vi "Command Drive Time with IMU.vi"(2 "Robot System Functions In":T1, 3 "Startup":bool, 4 "String Parameter":string, 5 "Cmd Parameter 3":dbl, 6 "Cmd Parameter 2":dbl, 7 "Cmd Parameter 1":dbl) -> (0 "Robot System Functions Out":T1, 1 "Completed":bool)   [LabVIEW 2016]
uses:
  Subsystems/All Robot Commands.ctl
  Subsystems/Drive and Climb SS/Drive + Climb Commands 2017.ctl
  Subsystems/Gear Delivery SS/Gear Delivery Commands.ctl
  Subsystems/Conveyor and Shooter SS/Conveyor and Shooter Commands.ctl
  Subsystems/Ball Intake SS/Ball Intake Commands.ctl
  Command Execution State.ctl
  <vilib>/Rock Robotics/WPI/ThirdParty/Sensors/Pigeon IMU/CTRE_PigeonIMU_TareType.ctl
  <vilib>/Rock Robotics/WPI/ThirdParty/CanMotor/TalonSRX/WPI_CANTalonSRX_APIControlMode.ctl
  Global Variables/Refnum Names.vi
  Global Variables/Auto Drive Calibrations.vi
  Global Variables/Sensor Data.vi
panel:
  out "Right F":dbl
  out "Right D":dbl
  out "Right I":dbl
  out "Right P":dbl
  out "Left F":dbl
  out "Left D":dbl
  out "Left I":dbl
  out "Left P":dbl
  # "Sample robot\ncontrol output.\nReplace with \nactual teleop \ncontrol signal \nstructure."
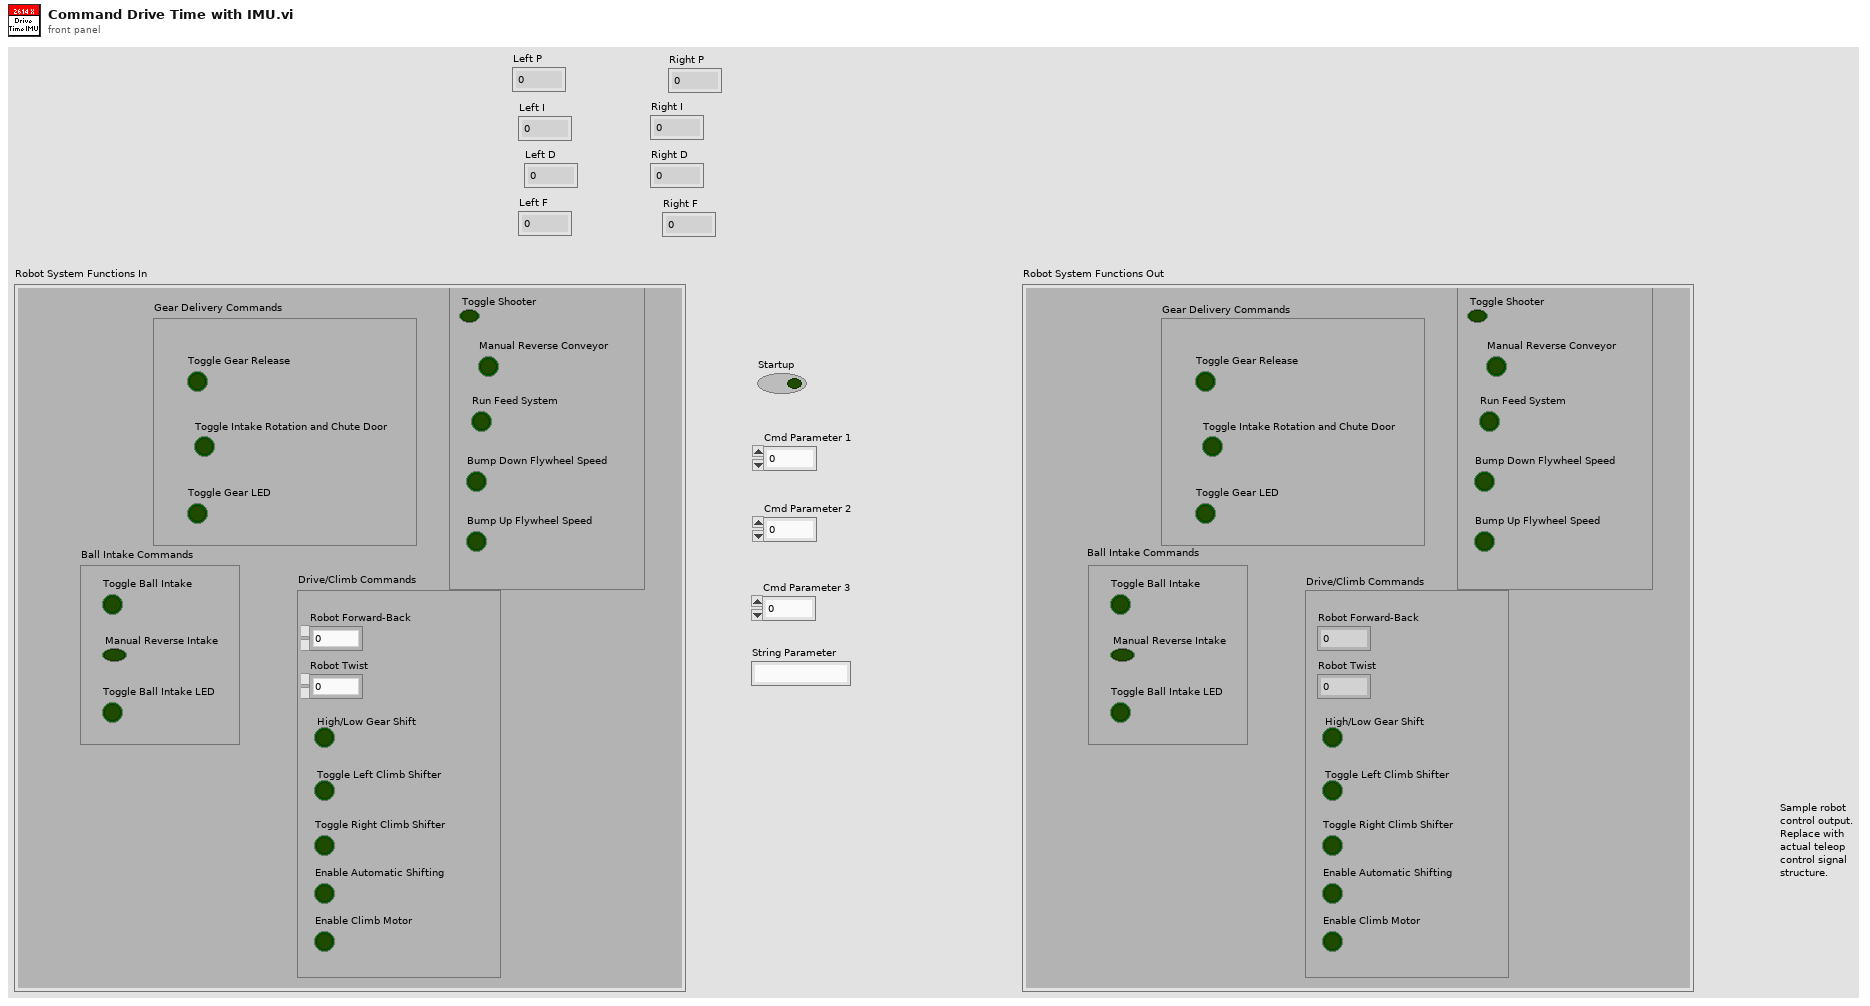
[diagram p1: front panel]
types:
  T1 = typedef "All Robot Commands.ctl" = cluster{"Drive/Climb Commands":T2, "Gear Delivery Commands":T3, "Shooter and Conveyor Commands":T4, "Ball Intake Commands":T5}
  T2 = typedef "Drive + Climb Commands 2017.ctl" = cluster{"Robot Forward-Back":dbl, "Robot Twist":dbl, "High/Low Gear Shift":bool, "Toggle Left Climb Shifter":bool, "Toggle Right Climb Shifter":bool, "Enable Automatic Shifting":bool, "Enable Climb Motor ":bool}
  T3 = typedef "Gear Delivery Commands.ctl" = cluster{"Toggle Gear Release":bool, "Toggle Intake Rotation and Chute Door":bool, "Toggle Gear LED":bool}
  T4 = typedef "Conveyor and Shooter Commands.ctl" = cluster{"Toggle Shooter":bool, "Manual Reverse Conveyor":bool, "Run Feed System":bool, "Bump Down Flywheel Speed":bool, "Bump Up Flywheel Speed":bool}
  T5 = typedef "Ball Intake Commands.ctl" = cluster{"Toggle Ball Intake":bool, "Manual Reverse Intake":bool, "Toggle Ball Intake LED":bool}
  T6 = typedef "Command Execution State.ctl" = enum16{"Initialize", "Execute", "Finish"}
  T7 = typedef "WPI_CANTalonSRX_APIControlMode.ctl" = enum8{"Percent VBus", "Speed", "Position", "Slave", "Unchanged / Invalid", "Voltage Compensation", "Current", "Motion Profile", "Motion Magic"}
  T8 = typedef "CTRE_PigeonIMU_TareType.ctl" = u8
  T9 = typedef "CTRE_PigeonIMU_DeviceRef.ctl" = cluster{"DeviceStatus":errorcluster, "Device Number":u8, "Type":T10, "Device ID":u32}
  T10 = typedef "CTRE_PigeonIMU_ConnectionType.ctl" = u32
  T11 = typedef "WPI_MotorControlDeviceRef.ctl" = cluster{"DeviceStatus":errorcluster, "Type":T12, "PWM":cluster{"PWM Channel":T13, "DeadBand":T14}, "CAN":cluster{"Device Number":u8, "SetOutput VI Ref":variant, "GetOutput VI Ref":variant, "Enable VI Ref":variant, "Disable VI Ref":variant, "Data":variant}, "Invert":bool}
  T12 = typedef "WPI_MotorControlType.ctl" = enum16{"PWM", "CAN"}
  T13 = typedef "FPGA_DIOPWMChannel.ctl" = enum8{"PWM 0", "PWM 1", "PWM 2", "PWM 3", "PWM 4", "PWM 5", "PWM 6", "PWM 7", "PWM 8", "PWM 9", "PWM MXP 0", "PWM MXP 1", "PWM MXP 2", "PWM MXP 3", "PWM MXP 4", "PWM MXP 5", "PWM MXP 6", "PWM MXP 7", "PWM MXP 8", "PWM MXP 9", "Invalid"}
  T14 = typedef "WPI_PWMDeadband.ctl" = cluster{"Name":string, "maxPositivePwm":i32, "minPositivePwm":i32, "centerPwm":i32, "maxNegativePwm":i32, "minNegativePwm":i32, "angularRange":u16}
  T15 = cluster{"Goal":dbl, "Process Variable":dbl, "Max Ouput":dbl, dbl, dbl, dbl, dbl}
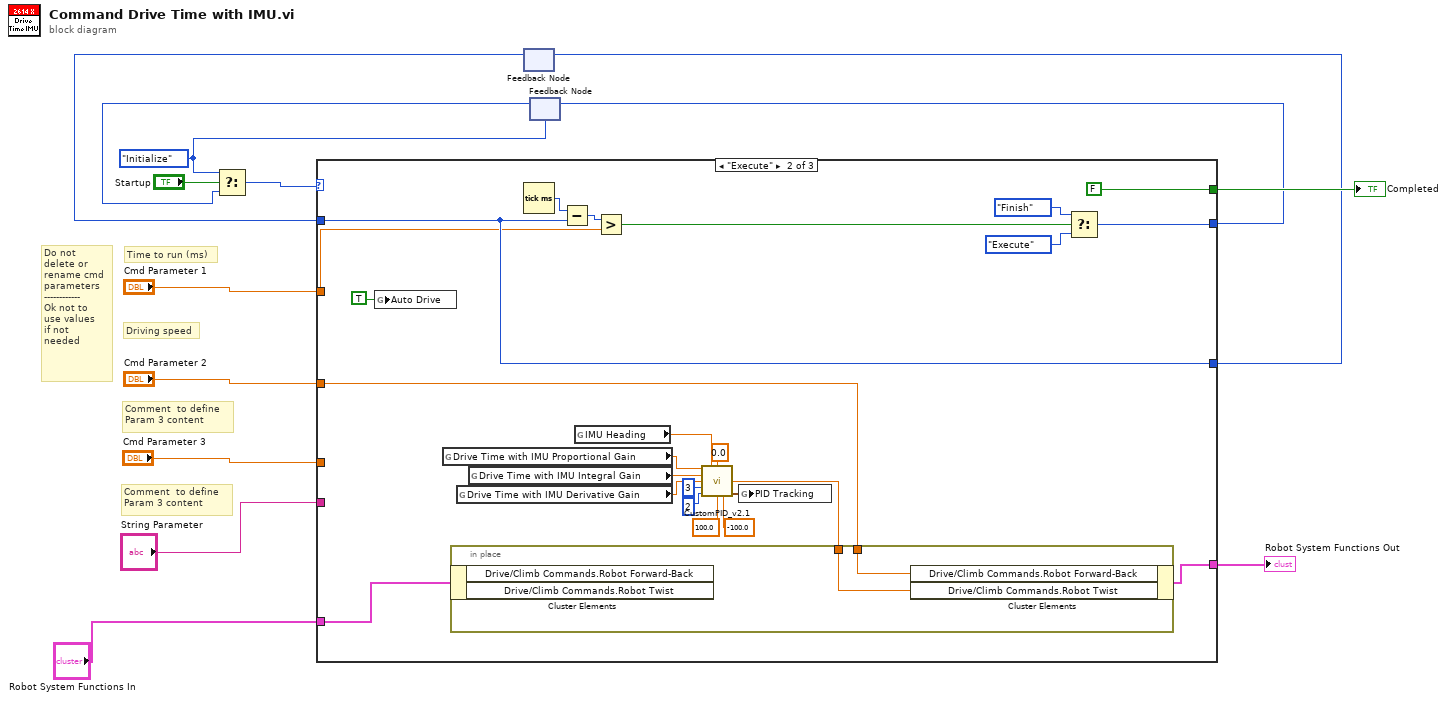
[diagram p0: block diagram]
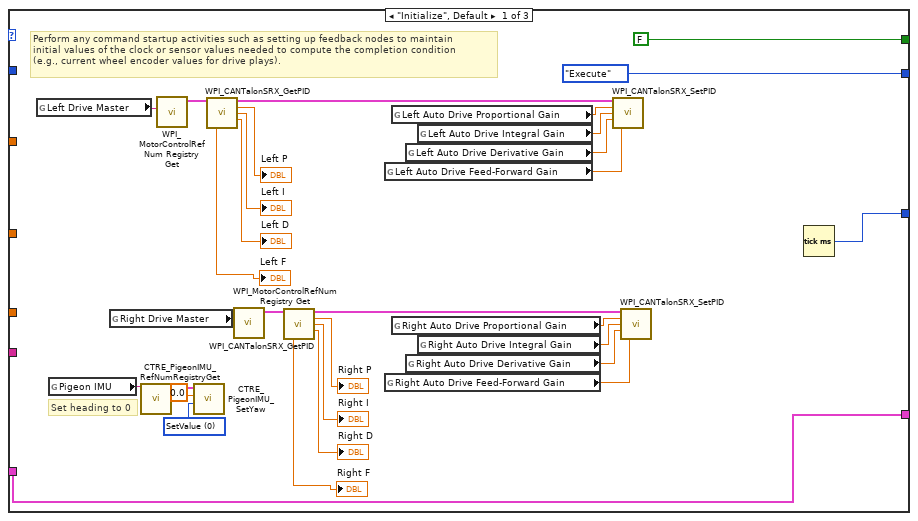
[diagram p2: hidden frame]
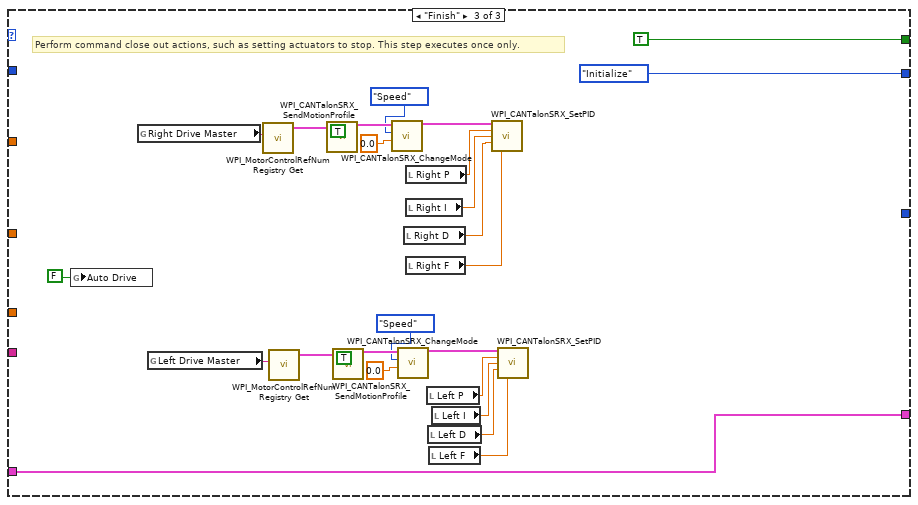
[diagram p3: hidden frame]
diagram:
  w9 = Command_Execution_State."Initialize" ("Play State")
  # "Comment  to define\nParam 3 content"
  # "Comment  to define\nParam 3 content"
  # "Do not \ndelete or\nrename cmd\nparameters\n------------\nOk not to \nuse values\nif not \nneeded"
  # "Driving speed"
  # "Time to run (ms)"
  n1 = feedback #1() -> (w1:u32)  [unwired: 1 in]
  n2 = feedback #2(w9) -> (w10:T6)
  n3 = Select(t=w9, s="Startup", f=w10) -> (s? t:f=w14:T6)
  n4 = case shown="\"Execute\"" w14 {
    tunnel: [FALSE FALSE TRUE] -> w12
    tunnel: [Command_Execution_State."Execute" ("Play State") w66 Command_Execution_State."Initialize" ("f")] -> w11
    tunnel: "Cmd Parameter 1" -> [_ w60 _]
    tunnel: "Cmd Parameter 2" -> [_ w45 _]
    tunnel: [w42 w58 w94] -> w6
    tunnel: "Robot System Functions In" -> [w42 w64 w94]
    tunnel: "Cmd Parameter 3" -> [_ _ _]
    tunnel: "String Parameter" -> [_ _ _]
    tunnel: [w41 w62 _] -> w2
    tunnel: w1 -> [_ w62 _]
    frame "Initialize", Default {
      w27 = T8 0 items=["SetValue"=0, "AddOffset"=1, "MatchCompass"=2, "SetOffset"=255] ("TareType (SetValue)")
      # "Set heading to 0"
      # "Perform any command startup activities such as setting up feedback nodes to maintain \ninitial values of the clock or sensor values needed to compute the completion condition\n(e.g., current wheel encoder values for drive plays)."
      n5 = global read "Refnum Names.vi" "Left Drive Master"() -> (w40:string)
      n6 = global read "Refnum Names.vi" "Pigeon IMU"() -> (w26:string)
      n7 = global read "Refnum Names.vi" "Right Drive Master"() -> (w34:string)
      n8 = call <vilib>:"CTRE_PigeonIMU_RefNumRegistryGet.vi"("refnum name"=w26) -> ("PigeonIMUDevRef"=w25:T9)  [unwired: 9 in, 1 out]
      n9 = call <vilib>:"WPI_MotorControlRefNum Registry Get.vi"("refnum name"=w40) -> ("MotorControlDevRef"=w39:T11)  [unwired: 9 in, 1 out]
      n10 = call <vilib>:"CTRE_PigeonIMU_SetYaw.vi"("TareType (SetValue)"=w27, "Value"=0.0, "PigeonIMUDevRef"=w25) -> ()  [unwired: 7 in, 2 out]
      n11 = call <vilib>:"WPI_CANTalonSRX_GetPID.vi"("CAN Talon SRX Ref"=w39) -> ("CAN Talon SRX Ref"=w15:T11, "P"=→"Left P":dbl, "I"=→"Left I":dbl, "D"=→"Left D":dbl, "F"=→"Left F":dbl)  [unwired: 7 in, 3 out]
      n12 = call <vilib>:"WPI_MotorControlRefNum Registry Get.vi"("refnum name"=w34) -> ("MotorControlDevRef"=w33:T11)  [unwired: 9 in, 1 out]
      n13 = call <vilib>:"WPI_CANTalonSRX_GetPID.vi"("CAN Talon SRX Ref"=w33) -> ("CAN Talon SRX Ref"=w16:T11, "P"=→"Right P":dbl, "I"=→"Right I":dbl, "D"=→"Right D":dbl, "F"=→"Right F":dbl)  [unwired: 7 in, 3 out]
      n14 = global read "Auto Drive Calibrations.vi" "Left Auto Drive Feed-Forward Gain"() -> (w17:dbl)
      n15 = global read "Auto Drive Calibrations.vi" "Right Auto Drive Feed-Forward Gain"() -> (w22:dbl)
      n16 = global read "Auto Drive Calibrations.vi" "Left Auto Drive Proportional Gain"() -> (w20:dbl)
      n17 = global read "Auto Drive Calibrations.vi" "Right Auto Drive Proportional Gain"() -> (w21:dbl)
      n18 = global read "Auto Drive Calibrations.vi" "Left Auto Drive Derivative Gain"() -> (w18:dbl)
      n19 = global read "Auto Drive Calibrations.vi" "Right Auto Drive Derivative Gain"() -> (w23:dbl)
      n20 = global read "Auto Drive Calibrations.vi" "Left Auto Drive Integral Gain"() -> (w19:dbl)
      n21 = global read "Auto Drive Calibrations.vi" "Right Auto Drive Integral Gain"() -> (w24:dbl)
      n22 = call <vilib>:"WPI_CANTalonSRX_SetPID.vi"("CAN Talon SRX Ref"=w15, "P"=w20, "I"=w19, "D"=w18, "F"=w17) -> ()  [unwired: 9 in, 2 out]
      n23 = call <vilib>:"WPI_CANTalonSRX_SetPID.vi"("CAN Talon SRX Ref"=w16, "P"=w21, "I"=w24, "D"=w23, "F"=w22) -> ()  [unwired: 9 in, 2 out]
      n24 = Tick Count (ms)() -> (millisecond timer value=w41:u32)
    }
    frame "Execute" {
      n25 = global write "Auto Drive Calibrations.vi" "Auto Drive"(TRUE ("PID Heading")) -> ()
      n26 = global read "Auto Drive Calibrations.vi" "Drive Time with IMU Proportional Gain"() -> (w50:dbl)
      n27 = global read "Auto Drive Calibrations.vi" "Drive Time with IMU Derivative Gain"() -> (w48:dbl)
      n28 = global read "Auto Drive Calibrations.vi" "Drive Time with IMU Integral Gain"() -> (w49:dbl)
      n29 = Tick Count (ms)() -> (millisecond timer value=w63:u32)
      n30 = Subtract(x=w63, y=w62) -> (x-y=w61:u32)
      n31 = global read "Sensor Data.vi" "IMU Heading"() -> (w47:dbl)
      n32 = Greater?(x=w61, y=w60) -> (0:w59:bool)
      n33 = call "CustomPID_v2.1.vi"("Kp"=w50, "Process Variable"=w47, "Goal"=0.0, "Ki"=w49, "Kd"=w48, "N-Diff"=3, "N-Int"=2, "Max Ouput"=100.0, "Min Output"=-100.0) -> ("Command"=w46:dbl, "PID Tracking"=w51:T15)  [unwired: 4 in, 1 out]
      n34 = in-place {
        in-place-border: w46 -> [w70]
        in-place-border: w45 -> [w69]
        n35 = in-place-cluster #3(w64) -> ()  [unwired: 2 out]
        n36 = in-place-cluster #3("Drive/Climb Commands.Robot Forward-Back"=w69, "Drive/Climb Commands.Robot Twist"=w70) -> (w58:T1)
      }
      n37 = global write "Auto Drive Calibrations.vi" "PID Tracking"(w51) -> ()
      n38 = Select(t=Command_Execution_State."Finish" ("Play State"), s=w59, f=Command_Execution_State."Execute") -> (s? t:f=w66:T6)
    }
    frame "Finish" {
      # "Perform command close out actions, such as setting actuators to stop. This step executes once only."
      n39 = global write "Auto Drive Calibrations.vi" "Auto Drive"(FALSE ("PID Heading")) -> ()
      n40 = global read "Refnum Names.vi" "Right Drive Master"() -> (w88:string)
      n41 = global read "Refnum Names.vi" "Left Drive Master"() -> (w77:string)
      n42 = call <vilib>:"WPI_MotorControlRefNum Registry Get.vi"("refnum name"=w88) -> ("MotorControlDevRef"=w93:T11)  [unwired: 9 in, 1 out]
      n43 = call <vilib>:"WPI_MotorControlRefNum Registry Get.vi"("refnum name"=w77) -> ("MotorControlDevRef"=w82:T11)  [unwired: 9 in, 1 out]
      n44 = call <vilib>:"WPI_CANTalonSRX_SendMotionProfile.vi"("CAN Talon SRX Ref"=w93, "Clear"=TRUE) -> ("CAN Talon SRX Ref Out"=w90:T11)  [unwired: 10 in, 3 out]
      n45 = call <vilib>:"WPI_CANTalonSRX_SendMotionProfile.vi"("CAN Talon SRX Ref"=w82, "Clear"=TRUE) -> ("CAN Talon SRX Ref Out"=w79:T11)  [unwired: 10 in, 3 out]
      n46 = call <vilib>:"WPI_CANTalonSRX_ChangeMode.vi"("Output"=0.0, "Control Mode"=WPI_CANTalonSRX_APIControlMode."Speed", "CAN Talon SRX Ref"=w90) -> ("CAN Talon SRX Ref"=w87:T11)  [unwired: 7 in, 1 out]
      n47 = call <vilib>:"WPI_CANTalonSRX_ChangeMode.vi"("Output"=0.0, "Control Mode"=WPI_CANTalonSRX_APIControlMode."Speed", "CAN Talon SRX Ref"=w79) -> ("CAN Talon SRX Ref"=w76:T11)  [unwired: 7 in, 1 out]
      n48 = local read "Right D"() -> (w84:dbl)
      n49 = local read "Right P"() -> (w86:dbl)
      n50 = local read "Right I"() -> (w85:dbl)
      n51 = local read "Right F"() -> (w83:dbl)
      n52 = local read "Left P"() -> (w75:dbl)
      n53 = local read "Left D"() -> (w73:dbl)
      n54 = local read "Left F"() -> (w72:dbl)
      n55 = local read "Left I"() -> (w74:dbl)
      n56 = call <vilib>:"WPI_CANTalonSRX_SetPID.vi"("CAN Talon SRX Ref"=w87, "P"=w86, "I"=w85, "D"=w84, "F"=w83) -> ()  [unwired: 9 in, 2 out]
      n57 = call <vilib>:"WPI_CANTalonSRX_SetPID.vi"("CAN Talon SRX Ref"=w76, "P"=w75, "I"=w74, "D"=w73, "F"=w72) -> ()  [unwired: 9 in, 2 out]
    }
  }
  "Completed" <- w12
  "Robot System Functions Out" <- w6
  n58 = feedback-in #1(w2) -> ()
  n59 = feedback-in #2(w11) -> ()
